vi "Stop.vi"(8 "error in (no error)":errorcluster, 10 "Message in":refnum<class "StopMessage.lvclass">, 11 "ImageStack in":refnum<class "Invivo_ImageStack.lvclass">) -> (0 "error out":errorcluster, 3 "ImageStack out":refnum<class "Invivo_ImageStack.lvclass">)   [LabVIEW 2012, in "Invivo_ImageStack.lvclass"]
doc: "This member function is called when the statemachine in the run.vi receives an 'stop' command. It relays the message to all observers of the component.\n\nOverride this member function in your derived class if you need additional stop functionality (but don't forget to call the parent method)."
uses:
  Invivo_ImageStack.lvclass
  <vilib>/Distrio/Murmex/StopMessage/StopMessage.lvclass
  <vilib>/Distrio/Murmex/GenericMessage/GenericMessage.lvclass
  <vilib>/Distrio/Murmex/Murmex/Murmex.lvclass
  Invivo_ImageStack.lvclass/Invivo_ImageStack.ctl
  <vilib>/Distrio/Murmex/Message/Add or replace parameter.vi
  <vilib>/Distrio/Murmex/Message/Message.lvclass
panel:
  # "This method is called when the STOP\ntrigger is sent. \n\nOverride this method when your component needs to\nrespond to this trigger. \n\nCall parent for proper implementation"
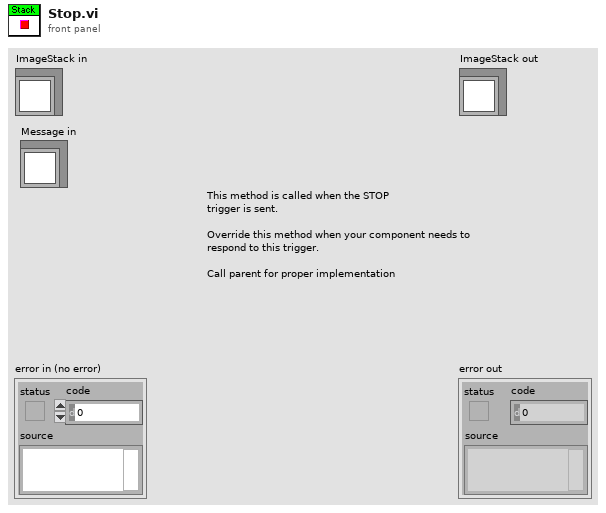
[diagram p1: front panel]
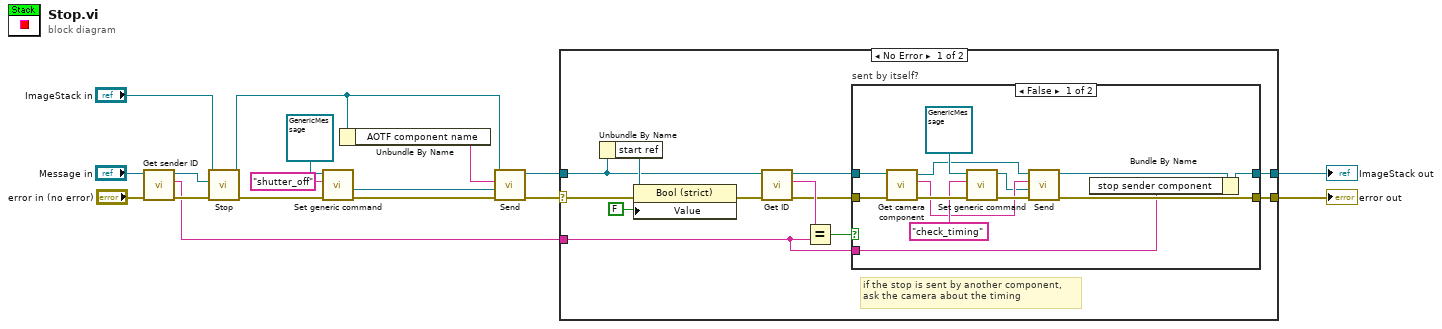
[diagram p0: block diagram]
diagram:
  n1 = call <vilib>:"Get sender ID.vi"("error in (no error)"="error in (no error)", "Message in"="Message in") -> ("error out"=w4:errorcluster, "sender"=w1:string, "Message out"=w2:refnum<class "StopMessage.lvclass">)  [unwired: 7 in]
  n2 = call-parent "Stop.vi"("error in (no error)"=w4, "Message in"=w2, "Murmex in"="ImageStack in") -> ("error out"=w10:errorcluster, "Murmex out"=w7:refnum<class "Invivo_ImageStack.lvclass">)  [unwired: 7 in]
  n3 = call <vilib>:"Set generic command.vi"("error in (no error)"=w10, "generic command"="shutter_off", "GenericMessage in"=refnum<class "GenericMessage.lvclass"> refnum ("Distrio Murmex 1.1:GenericMessage")) -> ("error out"=w14:errorcluster, "GenericMessage out"=w11:refnum<class "GenericMessage.lvclass">)  [unwired: 7 in]
  n4 = Unbundle By Name(w7) -> ("AOTF component name"=w6:string)
  n5 = call <vilib>:"Send.vi"("error in (no error)"=w14, "Message"=w11, "recipient"=w6, "Murmex in"=w7) -> ("error out"=w9:errorcluster, "Murmex out"=w8:refnum<class "Invivo_ImageStack.lvclass">)  [unwired: 6 in]
  n6 = case shown="No Error" w9 {
    selector: w9 -> [w27 w45]
    tunnel: w8 -> [w25 w46]
    tunnel: [w20 w45] -> w15
    tunnel: [w22 w46] -> w16
    tunnel: w1 -> [w18 _]
    frame No Error {
      # "if the stop is sent by another component,\nask the camera about the timing"
      n7 = Unbundle By Name(w25) -> ("start ref"=w28:refnum<vi>)
      n8 = property class="Bool (strict)"(reference=w28, error in=w27, "Value"=FALSE) -> (error out=w26:errorcluster)  [unwired: 1 out]
      n9 = call <vilib>:"Get ID.vi"("error in (no error)"=w26, "Murmex in"=w25) -> ("error out"=w19:errorcluster, "component id"=w24:string, "Murmex out"=w21:refnum<class "Invivo_ImageStack.lvclass">)  [unwired: 7 in]
      n10 = Equal?(x=w24, y=w18) -> (x = y?=w23:bool)
      n11 = case "sent by itself?" shown="False" w23 {
        tunnel: [w31 w44] -> w22
        tunnel: w21 -> [w42 w44]
        tunnel: [w36 w43] -> w20
        tunnel: w19 -> [w41 w43]
        tunnel: w18 -> [w30 _]
        frame False {
          n12 = call-dynamic "Get camera component.vi"("error in (no error)"=w41, "ImageStack in"=w42) -> ("error out"=w40:errorcluster, "Camera component name"=w35:string, "ImageStack out"=w34:refnum<class "Invivo_ImageStack.lvclass">)  [unwired: 7 in]
          n13 = call <vilib>:"Set generic command.vi"("error in (no error)"=w40, "generic command"="check_timing", "GenericMessage in"=refnum<class "GenericMessage.lvclass"> refnum ("Distrio Murmex 1.2:GenericMessage")) -> ("error out"=w37:errorcluster, "GenericMessage out"=w33:refnum<class "GenericMessage.lvclass">)  [unwired: 7 in]
          n14 = call <vilib>:"Send.vi"("error in (no error)"=w37, "Message"=w33, "recipient"=w35, "Murmex in"=w34) -> ("error out"=w36:errorcluster, "Murmex out"=w32:refnum<class "Invivo_ImageStack.lvclass">)  [unwired: 6 in]
          n15 = Bundle By Name(cluster=w32, "stop sender component"=w30) -> (w31:refnum<class "Invivo_ImageStack.lvclass">)
        }
        frame True {
        }
      }
    }
    frame Error {
    }
  }
  "error out" <- w15
  "ImageStack out" <- w16
